vi "JSON Config Boolean Vector.vi"(7 "Class":refnum<class "Abs_Boolean.lvclass">, 8 "error in (no error)":errorcluster, 11 "Test Value":bool) -> (0 "error out":errorcluster)   [LabVIEW 2021]
uses:
  Source/Abs_Types/Boolean/Abs_Boolean.lvclass
  C:/New folder/LV_Abstract/LV_Abstract/Source/Abs_Types/Type/Abs_Type.lvclass
  Source/Abs_Types/Boolean/Simple Read.vi
  Source/Constants/Support/Bool/Bool.vi
  <vilib>/addons/_JKI Toolkits/Caraya/classes/Assert/Assert Equal Value_Variant.vi
  <vilib>/addons/_JKI Toolkits/Caraya/classes/Assert/Assert Equal Type_Variant.vi
  <vilib>/addons/_JKI Toolkits/Caraya/classes/Assert/Assert.lvclass
  <vilib>/addons/_JKI Toolkits/Caraya/classes/Test/Test.lvclass
  <vilib>/Utility/Data Type/NI_Data Type.lvlib
  Source/Abs_Types/Type/Abs_Type.lvclass
  Source/Constants/Support/Bool/Const_Bool.lvclass
panel:
  out "JSON":string
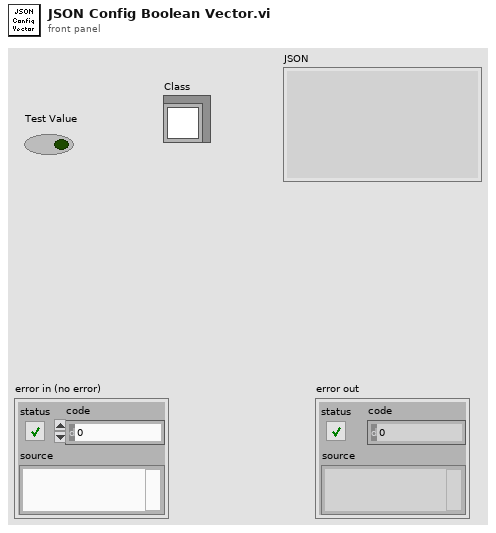
[diagram p1: front panel]
types:
  T1 = typedef "NI_Data Type.lvlib/Data Type.ctl" = enum8{"Invalid Type", "Void", "I8", "I16", "I32", "I64", "U8", "U16", "U32", "U64", "Single Float", "Double Float", "Extended Float", "Single Complex", "Double Complex", "Extended Complex", "Enum U8", "Enum U16", "Enum U32", "Enum U64", "Single Float With Unit", "Double Float With Unit", "Extended Float With Unit", "Single Complex with Unit", "Double Complex with Unit", "Extended Complex with Unit", "Boolean", "String", "Path", "Picture", "Tag", "Array", "Cluster", "Variant", "LV Variant", "Waveform", "Timestamp", "Digital Waveform", "Digital Data", "ExpressData", "Refnum", "External Data", "VI", "Poly VI", "LabVIEW Class Instance", "Fixed Point", "Set Collection", "Map Collection"}
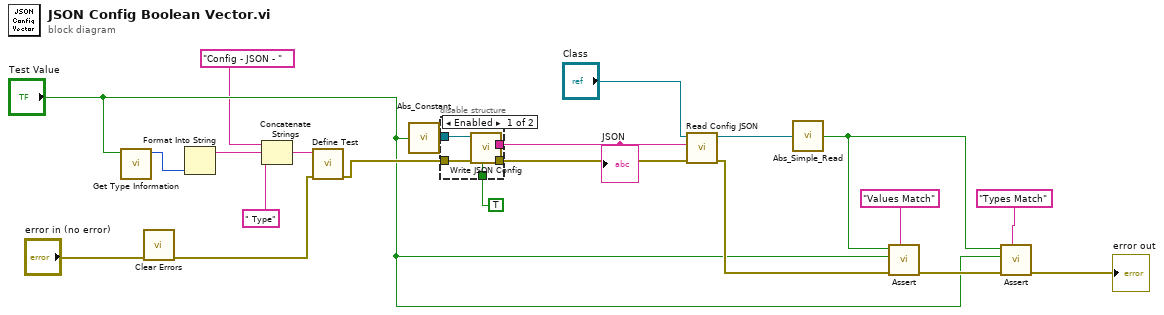
[diagram p0: block diagram]
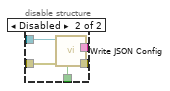
[diagram p2: hidden frame]
diagram:
  n1 = call <vilib>:"Get Type Information.vi"("variant"="Test Value") -> ("type"=w13:T1)  [unwired: 6 in, 4 out]
  n2 = call <vilib>:"Clear Errors.vi"("error in (no error)"="error in (no error)") -> ("error out"=w8:errorcluster)  [unwired: 5 in, 1 out]
  n3 = Format Into String(w13) -> (resulting string=w12:string)  [unwired: 3 in, 1 out]
  n4 = Concatenate Strings("Config - JSON - " ("string"), w12, " Type" ("string")) -> (w11:string)
  n5 = call <vilib>:"Define Test.vi"("error in (no error)"=w8, "Label (VI Title)"=w11) -> ("error out"=w14:errorcluster)  [unwired: 8 in, 1 out]
  n6 = call-poly "Abs_Constant.vi"("Boolean"="Test Value") -> ("Abs_Boolean.lvclass"=w21:refnum<class "Abs_Boolean.lvclass">)  [unwired: 4 in]
  n7 = disable-structure shown="Enabled" {
    disable-tunnel: w21 -> [w26 w31]
    disable-tunnel: TRUE ("Include Class Name") -> [w25 w30]
    disable-tunnel: [w24 w29] -> w19
    disable-tunnel: [w23 w28] -> w18
    disable-tunnel: w14 -> [w22 w27]
    frame Enabled {
      n8 = call-dynamic "Write JSON Config.vi"("Pretty Print?"=w25, "error in (no error)"=w22, "Abs_Type in"=w26) -> ("error out"=w23:errorcluster, "JSON"=w24:string)  [unwired: 6 in, 1 out]
    }
    frame Disabled {
      n9 = call-dynamic "Write JSON Config.vi"("Pretty Print?"=w30, "error in (no error)"=w27, "Abs_Type in"=w31) -> ("error out"=w28:errorcluster, "JSON"=w29:string)  [unwired: 6 in, 1 out]
    }
  }
  "JSON" <- w19
  n10 = call "Read Config JSON.vi"("error in (no error)"=w18, "JSON Config"=w19, "Abs_Type in"="Class") -> ("error out"=w16:errorcluster, "Abs_Type out"=w17:refnum<class "Abs_Boolean.lvclass">)  [unwired: 7 in]
  n11 = call-poly "Abs_Simple_Read.vi"("Boolean in"=w17) -> ("Boolean"=w5:bool)  [unwired: 4 in]
  n12 = call-poly <vilib>:"Assert.vi"("Label"="Values Match", "error in (no error)"=w16, "Actual"="Test Value", "Expected"=w5) -> ("error out"=w6:errorcluster)  [unwired: 6 in, 1 out]
  n13 = call-poly <vilib>:"Assert.vi"("Label"="Types Match", "error in (no error)"=w6, "Actual"="Test Value", "Expected"=w5) -> ("error out"=→"error out":errorcluster)  [unwired: 6 in, 1 out]
